vi "CCE MGLD PMJD PF SubVI01.vi"(11 "captura":T1) -> (0 "Image 4":T1(plugin-control), 1 "y":sgl, 2 "x":sgl, 3 "tapa detectada":bool)   [LabVIEW 2020]
doc: "Ceballos Conde Emanuel Meneses Gutiérrez Luis David Pineda Méndez Job Daniel 4MV6 Sistemas de visión artificial 2022/1 \nEste vi detecta si se encuentra o no una taparrosca en la imagen y devuelve las coordenadas en pixeles del centro de esta"
uses:
  <vilib>/vision/Image Controls.llb/IMAQ Image.ctl
  <vilib>/vision/NI_Vision_Development_Module.lvlib
panel:
  out "Image 2":T1(plugin-control)
  out "patron":T1(plugin-control)
  out "Matches (real-world)":T2(array[cluster]) {"Bounding Box"."y" format="%.2f"; "Bounding Box"."x" format="%.2f"; "Score" format="%.2f"; "Scale" format="%.2f"; "Angle" format="%.2f"; "Position"."y" format="%.2f"; "Position"."x" format="%.2f"}
  out "Number of Matches":i32
  # "Ceballos Conde Emanuel  Meneses Gutiérrez Luis David  Pineda Méndez Job Daniel 4MV6 Sistemas de visión artificial  2022/1             SubVI01"
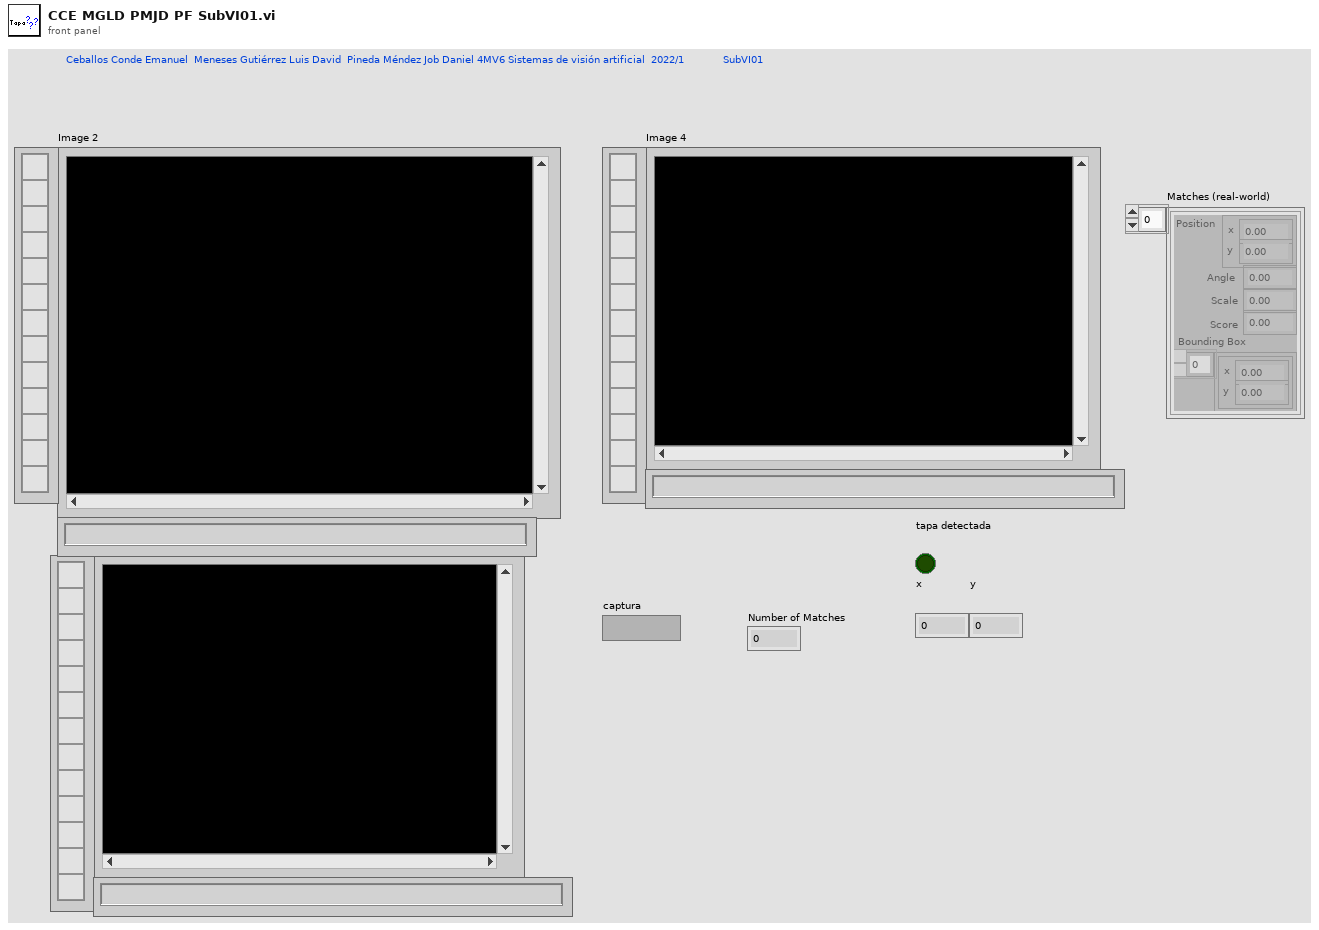
[diagram p1: front panel]
types:
  T1 = typedef "IMAQ Image.ctl" = refnum<image>
  T2 = cluster{"Position":cluster{"x":sgl, "y":sgl}, "Angle":sgl, "Scale":sgl, "Score":sgl, "Bounding Box":cluster{"x":sgl, "y":sgl}[]}[]
  T3 = cluster{"Number of Matches Requested":i32, "Minimum Match Score":sgl, "Angle Ranges":cluster{"Start Angle":sgl, "End Angle":sgl}[]}
  T4 = typedef "Image Type" = u32
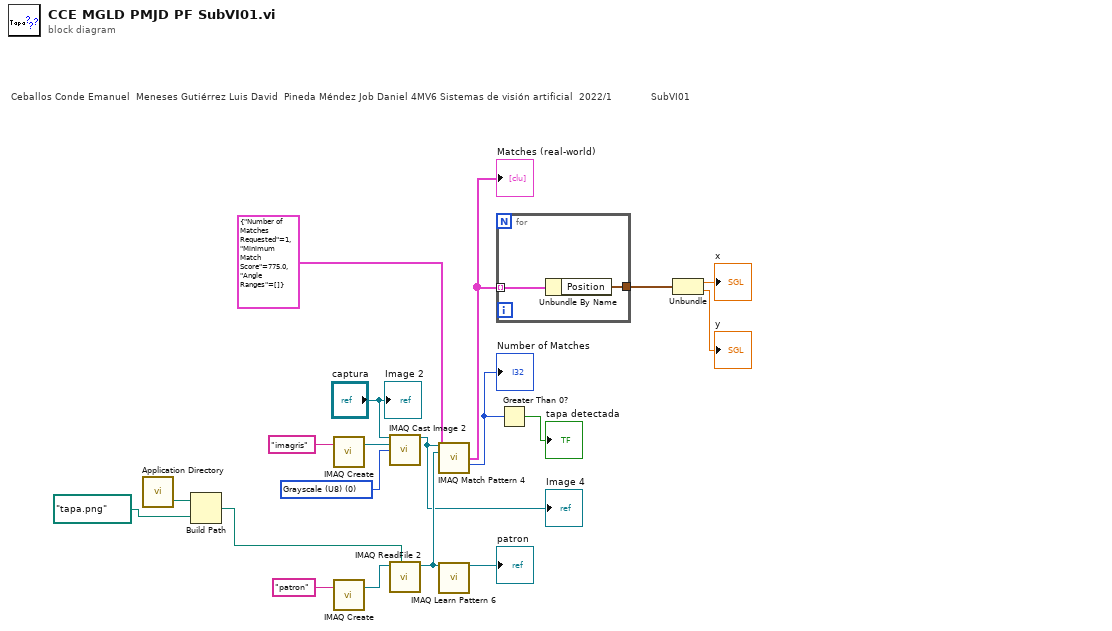
[diagram p0: block diagram]
diagram:
  w13 = T4 0 items=["Grayscale (U8)", "Grayscale (I16)", "Grayscale (SGL)", "Complex (CSG)", "RGB (U32)", "HSL (U32)", "RGB (U64)", "Grayscale (U16)"] ("Image Type")
  # "Ceballos Conde Emanuel  Meneses Gutiérrez Luis David  Pineda Méndez Job Daniel 4MV6 Sistemas de visión artificial  2022/1             SubVI01"
  n1 = call <vilib>:"Application Directory.vi"() -> ("Application Directory"=w3:path)
  n2 = Build Path(base path=w3, name or relative path=path "tapa.png") -> (appended path=w2:path)
  n3 = call "IMAQ Create"("Image Name"="imagris") -> ("New Image"=w15:T1)  [unwired: 4 in, 1 out]
  n4 = call "IMAQ Create"("Image Name"="patron") -> ("New Image"=w17:T1)  [unwired: 4 in, 1 out]
  n5 = call "IMAQ Cast Image 2"("Image Src"="captura", "Image Dst"=w15, "Image Type"=w13) -> ("Image Dst Out"=w5:T1)  [unwired: 11 in, 1 out]
  "Image 4" <- w5
  n6 = call "IMAQ ReadFile 2"("File Path"=w2, "Image"=w17) -> ("Image Out"=w16:T1)  [unwired: 5 in, 4 out]
  n7 = call "IMAQ Match Pattern 4"("Image"=w5, "Template Image"=w16, "Parameters"=T3 {"Number of Matches Requested"=1, "Minimum Match Score"=775.0, "Angle Ranges"=[]}) -> ("Matches (real-world)"=w12:T2, "Number of Matches"=w11:i32)  [unwired: 8 in, 3 out]
  "Matches (real-world)" <- w12
  "Number of Matches" <- w11
  n8 = call "IMAQ Learn Pattern 6"("Image"=w16) -> ("Template Image Out"=→"patron":T1)  [unwired: 12 in, 2 out]
  n9 = for {
    tunnel: w12 -> [w21] mode=indexing
    tunnel: [w20] -> w9
    n10 = Unbundle By Name(w21) -> ("Position"=w20:cluster{"x":sgl, "y":sgl})
  }
  n11 = Greater Than 0?(x=w11) -> (x > 0?=→"tapa detectada":bool)
  n12 = Unbundle(w9) -> ("x"=→"x":sgl, "y"=→"y":sgl)
  "Image 2" <- "captura"
